vi "Round_with_precision.vi"(1 "precision (6)":i16, 2 "number":dbl) -> (6 "rounded number":dbl)   [LabVIEW 2011]
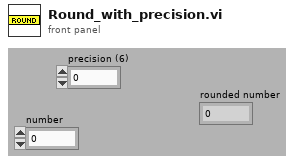
[diagram p1: front panel]
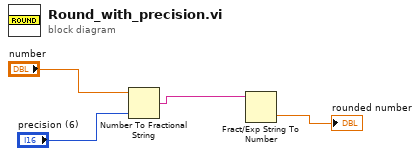
[diagram p0: block diagram]
diagram:
  n1 = Number To Fractional String(number="number", precision (6)="precision (6)") -> (F-format string=w2:string)  [unwired: 2 in]
  n2 = Fract/Exp String To Number(string=w2) -> (number=→"rounded number":dbl)  [unwired: 3 in, 1 out]
